vi "DELETE.vi"(8 "error in":errorcluster, 10 "httpRequest":refnum<class "httpRequest.lvclass">, 11 "http-client in":refnum<class "httpClient.lvclass">) -> (0 "error out":errorcluster, 2 "httpResponse":refnum<class "httpResponse.lvclass">, 3 "http-client out":refnum<class "httpClient.lvclass">)   [LabVIEW 2020, in "httpClient.lvlib" / "httpClient.lvclass"]
uses:
  httpClient.lvclass
  httpRequest/httpRequest.lvclass
  httpResponse/httpResponse.lvclass
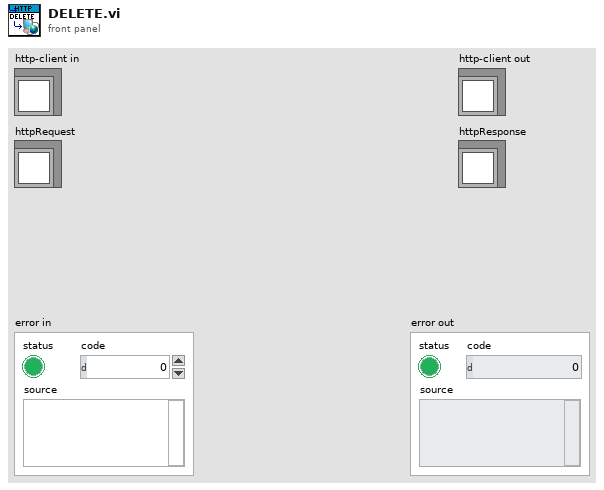
[diagram p1: front panel]
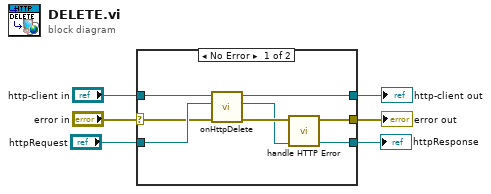
[diagram p0: block diagram]
diagram:
  n1 = case shown="No Error" "error in" {
    selector: "error in" -> [w12 w16]
    tunnel: [w9 w16] -> w5
    tunnel: [w11 w15] -> w3
    tunnel: "http-client in" -> [w14 w15]
    tunnel: [w8 _] -> w2
    tunnel: "httpRequest" -> [w13 _]
    frame No Error {
      n2 = call-dynamic "onHttpDelete.vi"("error in"=w12, "httpRequest"=w13, "http-method in"=w14) -> ("error out"=w10:errorcluster, "httpResponse"=w7:refnum<class "httpResponse.lvclass">, "http-method out"=w11:refnum<class "httpClient.lvclass">)  [unwired: 6 in]
      n3 = call "handle HTTP Error.vi"("httpResponse"=w7, "error in (no error)"=w10) -> ("httpResponse out"=w8:refnum<class "httpResponse.lvclass">, "error out"=w9:errorcluster)  [unwired: 8 in]
    }
    frame Error {
    }
  }
  "error out" <- w5
  "http-client out" <- w3
  "httpResponse" <- w2
